vi "Comm@Connect__Parameter.vi"(1 "ParamterIn":string) -> (0 "ParamterOut":string)   [LabVIEW 2019]
panel:
  in  "ID":string(combo)="1"
  in  "COM_Setting":string(combo)
  in  "COM_BaudRate":string(combo)
  in  "Control":string(combo)
  in  "Message":string(combo)
  in  "Terminater":string(combo)
  in  "Ascii/Binary":string(combo)
  in  "CommName":string(combo)
  in  "Confirm":bool
  in  "Tab Control":T1(tab)
  # "Comm@Connect $Comm,$Type,$Parameter"
  # "COM               $Com,19200,{7,8}{N,E,O}{1,1.5,2},{Ascii,Binary}(,Terminater)\nTCP                $IP:$Port,{Ascii,Binary}(,Terminater)\nServer            $Port,{Ascii,Binary}(,Terminater)\nModbus           $Com,$ID,19200,{8,7}{N,E,O}{1,1.5,2},{Ascii,Binary}\nModbus(TCP)   $IP:$Port"
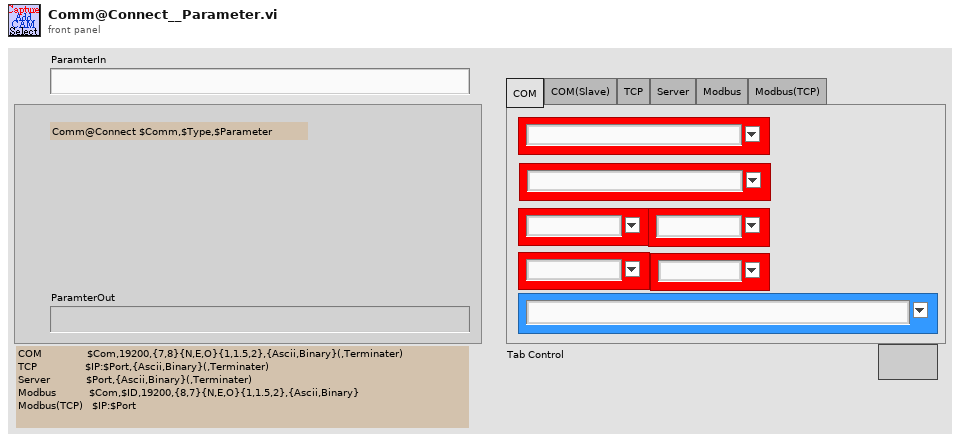
[diagram p1: front panel]
types:
  T1 = enum32{"COM", "COM(Slave)", "TCP", "Server", "Modbus", "Modbus(TCP)"}
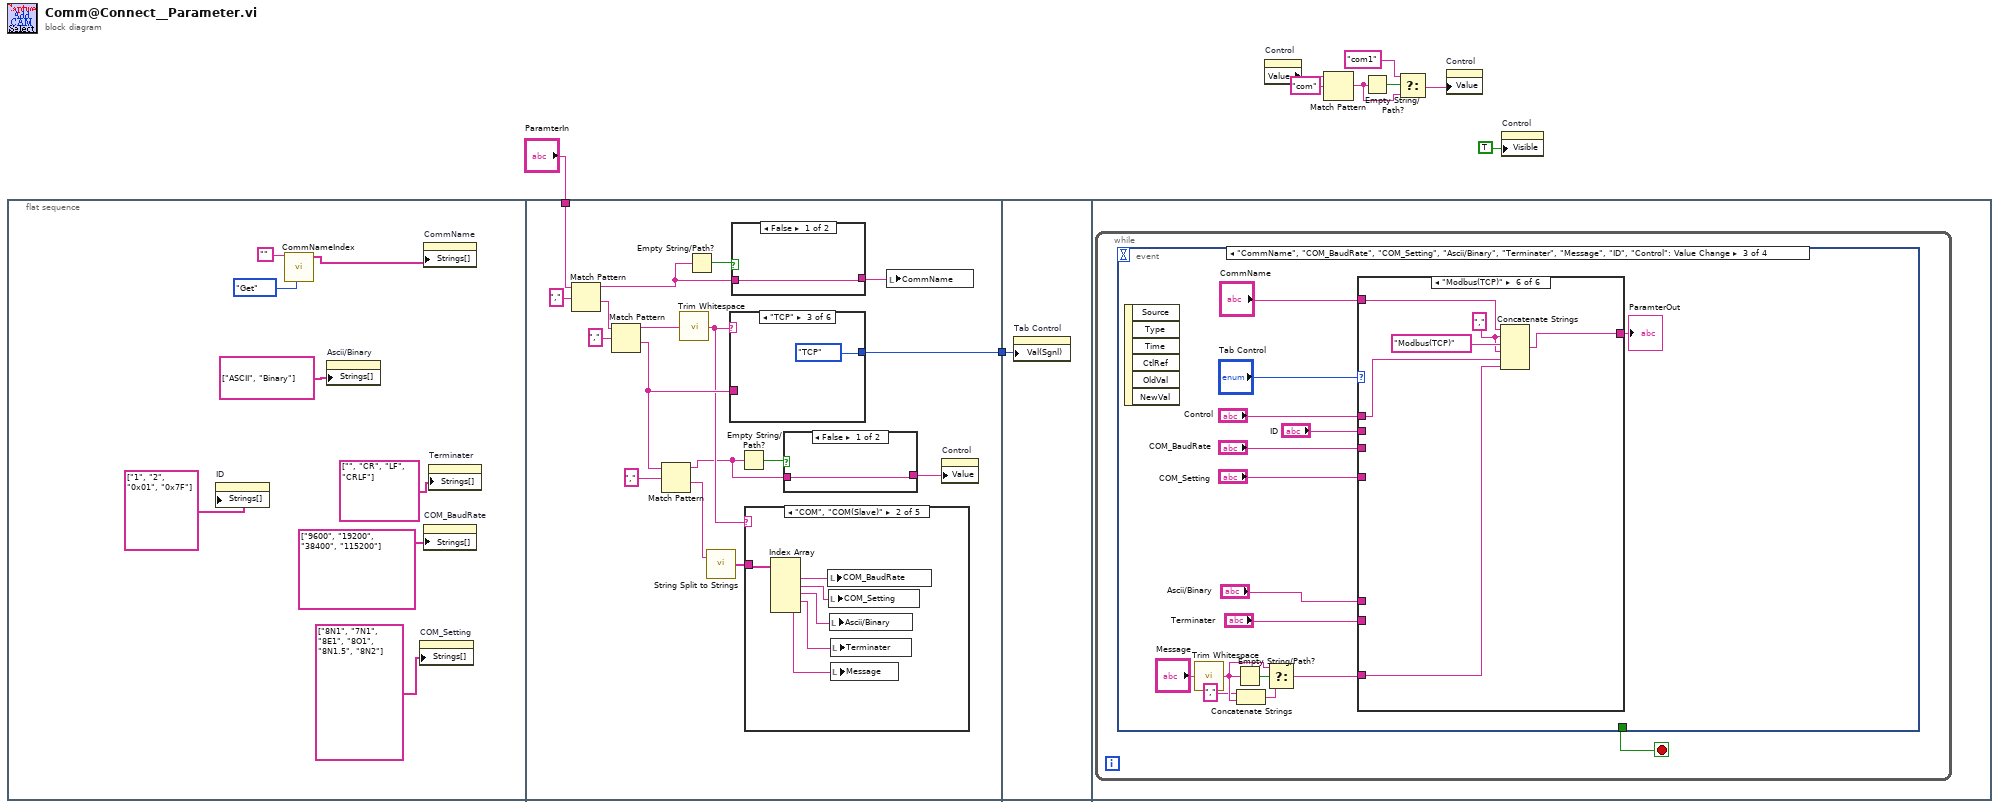
[diagram p0: block diagram]
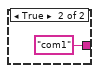
[diagram p2: hidden frame]
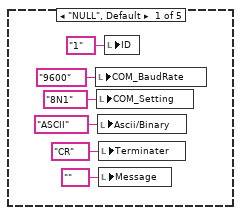
[diagram p3: hidden frame]
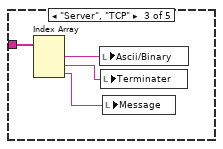
[diagram p4: hidden frame]
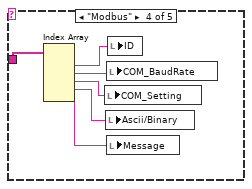
[diagram p5: hidden frame]
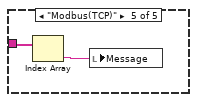
[diagram p6: hidden frame]
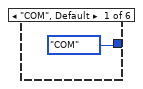
[diagram p7: hidden frame]
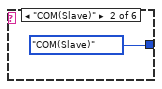
[diagram p8: hidden frame]
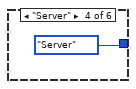
[diagram p9: hidden frame]
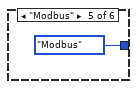
[diagram p10: hidden frame]
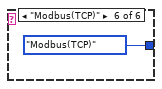
[diagram p11: hidden frame]
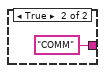
[diagram p12: hidden frame]
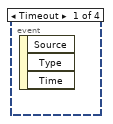
[diagram p13: hidden frame]
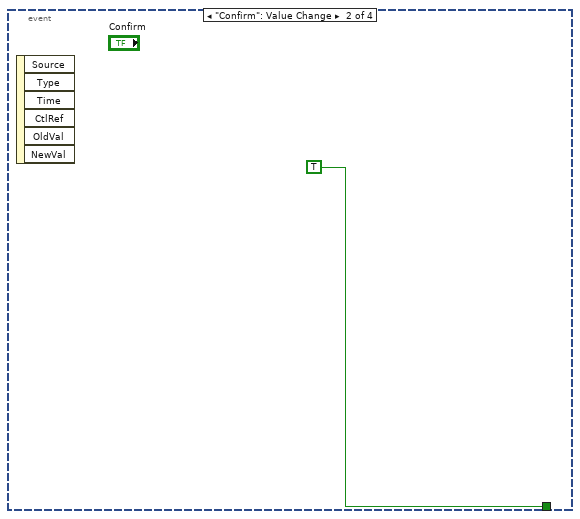
[diagram p14: hidden frame]
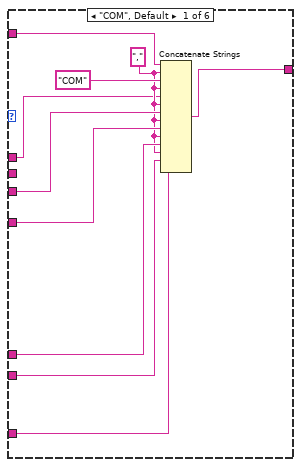
[diagram p15: hidden frame]
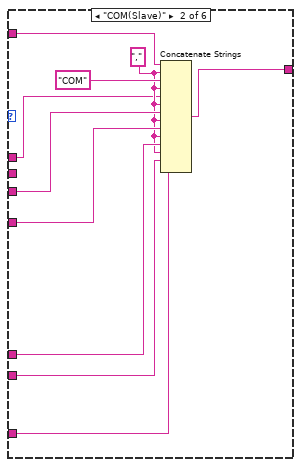
[diagram p16: hidden frame]
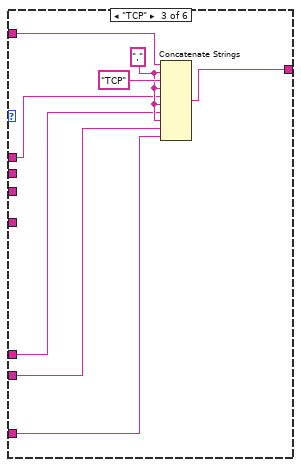
[diagram p17: hidden frame]
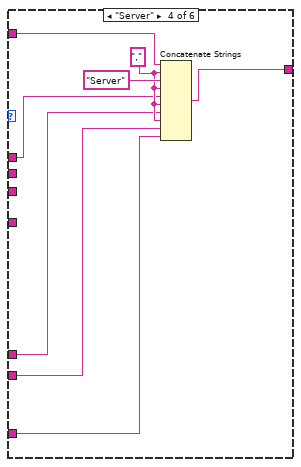
[diagram p18: hidden frame]
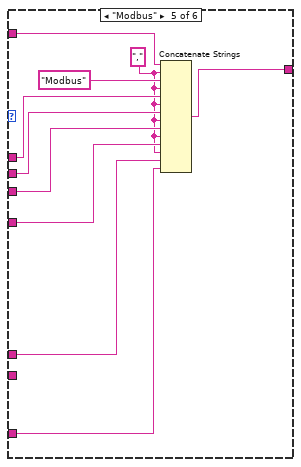
[diagram p19: hidden frame]
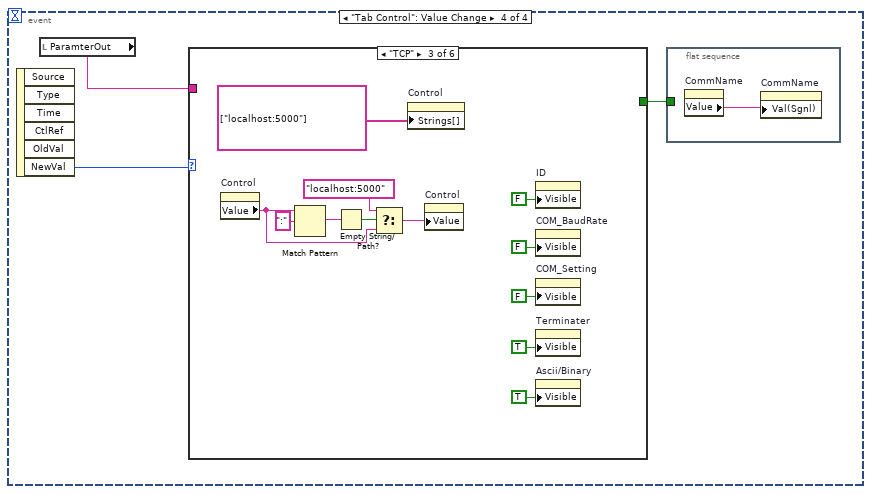
[diagram p20: hidden frame]
diagram:
  n1 = flat-sequence {
    tunnel: "ParamterIn" -> [w27]
    tunnel: [w26] -> w8
    tunnel: w8 -> [w69]
    frame #0 {
      n2 = property on="ID" class="CmbBox"("Strings[]"=string[] ["1", "2", "0x01", "0x7F"] ("Strings []")) -> ()  [unwired: 2 in, 2 out]
      n3 = call "CommNameIndex.vi"("OP"=enum16{"Init", "Get", "Set"}."Get", "Comm"="") -> ("CommNameS"=w15:string[])  [unwired: 7 in, 2 out]
      n4 = property on="Ascii/Binary" class="CmbBox"("Strings[]"=string[] ["ASCII", "Binary"] ("Strings []")) -> ()  [unwired: 2 in, 2 out]
      n5 = property on="COM_Setting" class="CmbBox"("Strings[]"=string[] ["8N1", "7N1", "8E1", "8O1", "8N1.5", "8N2"] ("Strings []")) -> ()  [unwired: 2 in, 2 out]
      n6 = property on="CommName" class="CmbBox"("Strings[]"=w15) -> ()  [unwired: 2 in, 2 out]
      n7 = property on="COM_BaudRate" class="CmbBox"("Strings[]"=string[] ["9600", "19200", "38400", "115200"] ("Strings []")) -> ()  [unwired: 2 in, 2 out]
      n8 = property on="Terminater" class="CmbBox"("Strings[]"=string[] ["", "CR", "LF", "CRLF"] ("Strings []")) -> ()  [unwired: 2 in, 2 out]
    }
    frame #1 {
      n9 = Match Pattern(string=w27, regular expression=",") -> (before substring=w30:string, after substring=w32:string)  [unwired: 1 in, 2 out]
      n10 = Match Pattern(string=w32, regular expression=",") -> (before substring=w29:string, after substring=w24:string)  [unwired: 1 in, 2 out]
      n11 = Match Pattern(string=w24, regular expression=",") -> (before substring=w19:string, after substring=w23:string)  [unwired: 1 in, 2 out]
      n12 = call <vilib>:"Trim Whitespace.vi"("string"=w29) -> ("trimmed string"=w22:string)  [unwired: 1 in]
      n13 = Empty String/Path?(string/path=w30) -> (empty?=w34:bool)
      n14 = call "String Split to Strings.vi"("String"=w23) -> ("Array"=w21:string[])  [unwired: 1 in]
      n15 = case shown="\"TCP\"" w22 {
        tunnel: [T1."COM" ("Tab Control") T1."COM(Slave)" ("Tab Control") T1."TCP" ("Tab Control") T1."Server" ("Tab Control") T1."Modbus" ("Tab Control") T1."Modbus(TCP)" ("Tab Control")] -> w26
        tunnel: w24 -> [_ _ _ _ _ _]
        frame "COM", Default {
        }
        frame "COM(Slave)" {
        }
        frame "TCP" {
        }
        frame "Server" {
        }
        frame "Modbus" {
        }
        frame "Modbus(TCP)" {
        }
      }
      n16 = case shown="False" w34 {
        tunnel: [w67 "COMM" ("ParamterIn")] -> w28
        tunnel: w30 -> [w67 _]
        frame False {
        }
        frame True {
        }
      }
      n17 = Empty String/Path?(string/path=w19) -> (empty?=w20:bool)
      n18 = case shown="\"COM\", \"COM(Slave)\"" w22 {
        tunnel: w21 -> [_ w48 w52 w56 w60]
        frame "NULL", Default {
          n19 = local write "COM_BaudRate"("9600" ("COM_BaudRate")) -> ()
          n20 = local write "COM_Setting"("8N1" ("COM_Setting")) -> ()
          n21 = local write "Ascii/Binary"("ASCII" ("Ascii/Binary")) -> ()
          n22 = local write "Terminater"("CR" ("Terminater")) -> ()
          n23 = local write "Message"("" ("Message")) -> ()
          n24 = local write "ID"("1" ("ID")) -> ()
        }
        frame "COM", "COM(Slave)" {
          n25 = Index Array(array=w48) -> (element #1=w47:string, element #2=w46:string, element #3=w45:string, element #4=w44:string, element #5=w43:string)  [unwired: 5 in]
          n26 = local write "COM_BaudRate"(w47) -> ()
          n27 = local write "COM_Setting"(w46) -> ()
          n28 = local write "Ascii/Binary"(w45) -> ()
          n29 = local write "Terminater"(w44) -> ()
          n30 = local write "Message"(w43) -> ()
        }
        frame "Server", "TCP" {
          n31 = Index Array(array=w52) -> (element #1=w51:string, element #2=w50:string, element #3=w49:string)  [unwired: 3 in]
          n32 = local write "Ascii/Binary"(w51) -> ()
          n33 = local write "Terminater"(w50) -> ()
          n34 = local write "Message"(w49) -> ()
        }
        frame "Modbus" {
          n35 = Index Array(array=w56) -> (element #1=w54:string, element #2=w55:string, element #3=w58:string, element #4=w57:string, element #5=w53:string)  [unwired: 5 in]
          n36 = local write "COM_Setting"(w58) -> ()
          n37 = local write "Ascii/Binary"(w57) -> ()
          n38 = local write "COM_BaudRate"(w55) -> ()
          n39 = local write "Message"(w53) -> ()
          n40 = local write "ID"(w54) -> ()
        }
        frame "Modbus(TCP)" {
          n41 = Index Array(array=w60) -> (element=w59:string)  [unwired: 1 in]
          n42 = local write "Message"(w59) -> ()
        }
      }
      n43 = case shown="False" w20 {
        tunnel: [w35 "com1" ("ParamterIn")] -> w18
        tunnel: w19 -> [w35 _]
        frame False {
        }
        frame True {
        }
      }
      n44 = local write "CommName"(w28) -> ()
      n45 = property on="Control" class="CmbBox"("Value"=w18) -> ()  [unwired: 2 in, 2 out]
    }
    frame #2 {
      n46 = property on="Tab Control" class="TabCtl (strict)"("Val(Sgnl)"=w69) -> ()  [unwired: 2 in, 2 out]
    }
    frame #3 {
      n47 = while {
        stop <- w70 stop-if-true
        n48 = event shown="[2] \"CommName\", \"COM_BaudRate\", \"COM_Setting\", \"Ascii/Binary\", \"Terminater\", \"Message\", \"ID\", \"Control\": Value Change" {
          selector: _ -> [_ _ _ _]
          dyn-events: _ -> [_ _ _ _]
          timeout: _ -> [_ _ _ _]
          tunnel: [_ TRUE _ _] -> w70
          event Timeout {
            n49 = event-data() -> ()  [unwired: 1 in, 3 out]
          }
          event "Confirm": Value Change {
            n50 = event-data() -> ()  [unwired: 1 in, 6 out]
          }
          event "CommName", "COM_BaudRate", "COM_Setting", "Ascii/Binary", "Terminater", "Message", "ID", "Control": Value Change {
            n51 = event-data() -> ()  [unwired: 1 in, 6 out]
            n52 = call <vilib>:"Trim Whitespace.vi"("string"="Message") -> ("trimmed string"=w80:string)  [unwired: 1 in]
            n53 = Empty String/Path?(string/path=w80) -> (empty?=w82:bool)
            n54 = Concatenate Strings("," ("string"), w80) -> (w81:string)
            n55 = Select(t=w80, s=w82, f=w81) -> (s? t:f=w78:string)
            n56 = case shown="\"Modbus(TCP)\"" "Tab Control" {
              tunnel: "CommName" -> [w96 w106 w114 w122 w132 w138]
              tunnel: [w94 w104 w112 w120 w130 w136] -> w84
              tunnel: w78 -> [w93 w103 w108 w116 w123 w133]
              tunnel: "Ascii/Binary" -> [w92 w102 w110 w118 w124 _]
              tunnel: "Terminater" -> [w91 w101 w109 w117 _ _]
              tunnel: "COM_BaudRate" -> [w89 w99 _ _ w128 _]
              tunnel: "COM_Setting" -> [w90 w100 _ _ w129 _]
              tunnel: "Control" -> [w87 w97 w107 w115 w127 w134]
              tunnel: "ID" -> [_ _ _ _ w126 _]
              frame "COM", Default {
                w88 = "," ("string")
                n57 = Concatenate Strings(w96, w88, "COM" ("string"), w88, w87, w88, w89, w88, w90, w88, w92, w88, w91, w93) -> (w94:string)
              }
              frame "COM(Slave)" {
                w98 = "," ("string")
                n58 = Concatenate Strings(w106, w98, "COM" ("string"), w98, w97, w98, w99, w98, w100, w98, w102, w98, w101, w103) -> (w104:string)
              }
              frame "TCP" {
                w111 = "," ("string")
                n59 = Concatenate Strings(w114, w111, "TCP" ("string"), w111, w107, w111, w110, w111, w109, w108) -> (w112:string)
              }
              frame "Server" {
                w119 = "," ("string")
                n60 = Concatenate Strings(w122, w119, "Server" ("string"), w119, w115, w119, w118, w119, w117, w116) -> (w120:string)
              }
              frame "Modbus" {
                w125 = "," ("string")
                n61 = Concatenate Strings(w132, w125, "Modbus" ("string"), w125, w127, w125, w126, w125, w128, w125, w129, w125, w124, w123) -> (w130:string)
              }
              frame "Modbus(TCP)" {
                w135 = "," ("string")
                n62 = Concatenate Strings(w138, w135, "Modbus(TCP)" ("string"), w135, w134, w133) -> (w136:string)
              }
            }
            "ParamterOut" <- w84
          }
          event "Tab Control": Value Change {
            n63 = event-data() -> ("NewVal"=w141:T1)  [unwired: 1 in, 5 out]
            n64 = local read "ParamterOut"() -> (w140:string)
            n65 = case shown="\"TCP\"" w141 {
              tunnel: w140 -> [_ _ _ _ _ _]
              tunnel: [TRUE _ _ _ _ _] -> w139
              frame "COM", Default {
                n66 = property on="Control" class="CmbBox"() -> ("Value"=w143:string)  [unwired: 2 in, 2 out]
                n67 = Match Pattern(string=w143, regular expression="com") -> (match substring=w144:string)  [unwired: 1 in, 3 out]
                n68 = Empty String/Path?(string/path=w144) -> (empty?=w147:bool)
                n69 = property on="Control" class="CmbBox"("Strings[]"=string[] ["com1", "com2", "com3"] ("Strings []")) -> ()  [unwired: 2 in, 2 out]
                n70 = Select(t="com1" ("f"), s=w147, f=w143) -> (s? t:f=w146:string)
                n71 = property on="Control" class="CmbBox"("Value"=w146) -> ()  [unwired: 2 in, 2 out]
                n72 = property on="ID" class="CmbBox"("Visible"=FALSE) -> ()  [unwired: 2 in, 2 out]
                n73 = property on="COM_BaudRate" class="CmbBox"("Visible"=TRUE) -> ()  [unwired: 2 in, 2 out]
                n74 = property on="COM_Setting" class="CmbBox"("Visible"=TRUE) -> ()  [unwired: 2 in, 2 out]
                n75 = property on="Terminater" class="CmbBox"("Visible"=TRUE) -> ()  [unwired: 2 in, 2 out]
                n76 = property on="Ascii/Binary" class="CmbBox"("Visible"=TRUE) -> ()  [unwired: 2 in, 2 out]
              }
              frame "COM(Slave)" {
                n77 = property on="Control" class="CmbBox"() -> ("Value"=w156:string)  [unwired: 2 in, 2 out]
                n78 = Match Pattern(string=w156, regular expression="com") -> (match substring=w157:string)  [unwired: 1 in, 3 out]
                n79 = property on="Control" class="CmbBox"("Strings[]"=string[] ["com1", "com2", "com3"] ("Strings []")) -> ()  [unwired: 2 in, 2 out]
                n80 = Empty String/Path?(string/path=w157) -> (empty?=w160:bool)
                n81 = Select(t="com1" ("f"), s=w160, f=w156) -> (s? t:f=w159:string)
                n82 = property on="Control" class="CmbBox"("Value"=w159) -> ()  [unwired: 2 in, 2 out]
                n83 = property on="ID" class="CmbBox"("Visible"=FALSE) -> ()  [unwired: 2 in, 2 out]
                n84 = property on="COM_BaudRate" class="CmbBox"("Visible"=TRUE) -> ()  [unwired: 2 in, 2 out]
                n85 = property on="COM_Setting" class="CmbBox"("Visible"=TRUE) -> ()  [unwired: 2 in, 2 out]
                n86 = property on="Terminater" class="CmbBox"("Visible"=TRUE) -> ()  [unwired: 2 in, 2 out]
                n87 = property on="Ascii/Binary" class="CmbBox"("Visible"=TRUE) -> ()  [unwired: 2 in, 2 out]
              }
              frame "TCP" {
                n88 = property on="Control" class="CmbBox"() -> ("Value"=w169:string)  [unwired: 2 in, 2 out]
                n89 = Match Pattern(string=w169, regular expression=":") -> (match substring=w170:string)  [unwired: 1 in, 3 out]
                n90 = Empty String/Path?(string/path=w170) -> (empty?=w172:bool)
                n91 = Select(t="localhost:5000", s=w172, f=w169) -> (s? t:f=w168:string)
                n92 = property on="Control" class="CmbBox"("Strings[]"=string[] ["localhost:5000"] ("Strings []")) -> ()  [unwired: 2 in, 2 out]
                n93 = property on="Control" class="CmbBox"("Value"=w168) -> ()  [unwired: 2 in, 2 out]
                n94 = property on="ID" class="CmbBox"("Visible"=FALSE) -> ()  [unwired: 2 in, 2 out]
                n95 = property on="COM_BaudRate" class="CmbBox"("Visible"=FALSE) -> ()  [unwired: 2 in, 2 out]
                n96 = property on="COM_Setting" class="CmbBox"("Visible"=FALSE) -> ()  [unwired: 2 in, 2 out]
                n97 = property on="Terminater" class="CmbBox"("Visible"=TRUE) -> ()  [unwired: 2 in, 2 out]
                n98 = property on="Ascii/Binary" class="CmbBox"("Visible"=TRUE) -> ()  [unwired: 2 in, 2 out]
              }
              frame "Server" {
                n99 = property on="Control" class="CmbBox"() -> ("Value"=w180:string)  [unwired: 2 in, 2 out]
                n100 = Match Pattern(string=w180, regular expression=":") -> (match substring=w182:string)  [unwired: 1 in, 3 out]
                n101 = Empty String/Path?(string/path=w182) -> (empty?=w184:bool)
                n102 = Select(t="*:5000", s=w184, f=w180) -> (s? t:f=w181:string)
                n103 = property on="Control" class="CmbBox"("Value"=w181) -> ()  [unwired: 2 in, 2 out]
                n104 = property on="Control" class="CmbBox"("Strings[]"=string[] ["*:5000"] ("Strings []")) -> ()  [unwired: 2 in, 2 out]
                n105 = property on="ID" class="CmbBox"("Visible"=FALSE) -> ()  [unwired: 2 in, 2 out]
                n106 = property on="COM_BaudRate" class="CmbBox"("Visible"=FALSE) -> ()  [unwired: 2 in, 2 out]
                n107 = property on="COM_Setting" class="CmbBox"("Visible"=FALSE) -> ()  [unwired: 2 in, 2 out]
                n108 = property on="Terminater" class="CmbBox"("Visible"=TRUE) -> ()  [unwired: 2 in, 2 out]
                n109 = property on="Ascii/Binary" class="CmbBox"("Visible"=TRUE) -> ()  [unwired: 2 in, 2 out]
              }
              frame "Modbus" {
                n110 = property on="Control" class="CmbBox"() -> ("Value"=w192:string)  [unwired: 2 in, 2 out]
                n111 = Match Pattern(string=w192, regular expression="com") -> (match substring=w193:string)  [unwired: 1 in, 3 out]
                n112 = Empty String/Path?(string/path=w193) -> (empty?=w196:bool)
                n113 = property on="Control" class="CmbBox"("Strings[]"=string[] ["com1", "com2", "com3"] ("Strings []")) -> ()  [unwired: 2 in, 2 out]
                n114 = Select(t="com1" ("f"), s=w196, f=w192) -> (s? t:f=w195:string)
                n115 = property on="Control" class="CmbBox"("Value"=w195) -> ()  [unwired: 2 in, 2 out]
                n116 = property on="ID" class="CmbBox"("Visible"=TRUE) -> ()  [unwired: 2 in, 2 out]
                n117 = property on="COM_BaudRate" class="CmbBox"("Visible"=TRUE) -> ()  [unwired: 2 in, 2 out]
                n118 = property on="COM_Setting" class="CmbBox"("Visible"=TRUE) -> ()  [unwired: 2 in, 2 out]
                n119 = property on="Terminater" class="CmbBox"("Visible"=FALSE) -> ()  [unwired: 2 in, 2 out]
                n120 = property on="Ascii/Binary" class="CmbBox"("Visible"=TRUE) -> ()  [unwired: 2 in, 2 out]
              }
              frame "Modbus(TCP)" {
                n121 = property on="Control" class="CmbBox"() -> ("Value"=w204:string)  [unwired: 2 in, 2 out]
                n122 = Match Pattern(string=w204, regular expression=":") -> (match substring=w206:string)  [unwired: 1 in, 3 out]
                n123 = Empty String/Path?(string/path=w206) -> (empty?=w208:bool)
                n124 = Select(t="localhost:5000", s=w208, f=w204) -> (s? t:f=w205:string)
                n125 = property on="Control" class="CmbBox"("Value"=w205) -> ()  [unwired: 2 in, 2 out]
                n126 = property on="Control" class="CmbBox"("Strings[]"=string[] ["localhost:5000"] ("Strings []")) -> ()  [unwired: 2 in, 2 out]
                n127 = property on="ID" class="CmbBox"("Visible"=FALSE) -> ()  [unwired: 2 in, 2 out]
                n128 = property on="COM_BaudRate" class="CmbBox"("Visible"=FALSE) -> ()  [unwired: 2 in, 2 out]
                n129 = property on="COM_Setting" class="CmbBox"("Visible"=FALSE) -> ()  [unwired: 2 in, 2 out]
                n130 = property on="Terminater" class="CmbBox"("Visible"=FALSE) -> ()  [unwired: 2 in, 2 out]
                n131 = property on="Ascii/Binary" class="CmbBox"("Visible"=FALSE) -> ()  [unwired: 2 in, 2 out]
              }
            }
            n132 = flat-sequence {
              tunnel: w139 -> [_]
              frame #0 {
                n133 = property on="CommName" class="CmbBox"() -> ("Value"=w142:string)  [unwired: 2 in, 2 out]
                n134 = property on="CommName" class="CmbBox"("Val(Sgnl)"=w142) -> ()  [unwired: 2 in, 2 out]
              }
            }
          }
        }
      }
    }
  }
  n135 = property on="Control" class="CmbBox"() -> ("Value"=w1:string)  [unwired: 2 in, 2 out]
  n136 = Match Pattern(string=w1, regular expression="com") -> (match substring=w6:string)  [unwired: 1 in, 3 out]
  n137 = Empty String/Path?(string/path=w6) -> (empty?=w3:bool)
  n138 = Select(t="com1" ("f"), s=w3, f=w6) -> (s? t:f=w4:string)
  n139 = property on="Control" class="CmbBox"("Value"=w4) -> ()  [unwired: 2 in, 2 out]
  n140 = property on="Control" class="CmbBox"("Visible"=TRUE) -> ()  [unwired: 2 in, 2 out]
